vi "energyDep.vi"(10 "B [T]":dbl, 11 "energy Dep in":dbl[](array[numeric])) -> (2 "Momentum [MeV/C]":dbl[](array[numeric]), 3 "energy dependence":dbl[](array[numeric]))   [LabVIEW 2020]
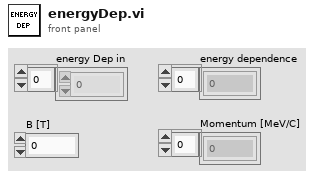
[diagram p1: front panel]
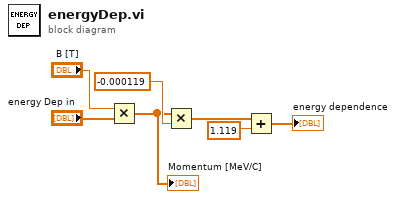
[diagram p0: block diagram]
diagram:
  n1 = Multiply(x="B [T]", y="energy Dep in") -> (x*y=w1:dbl[])
  "Momentum [MeV/C]" <- w1
  n2 = Multiply(x=w1, y=-0.000119) -> (x*y=w3:dbl[])
  n3 = Add(x=w3, y=1.119) -> (x+y=→"energy dependence":dbl[])
